vi "openMotor.vi"(3 "S/N Motor":string(combo)) -> (0 "Device":refnum<k24>, 1 ".NET Refnum out":refnum<k24>)   [LabVIEW 2014]
doc: "André Romero\nandretec@ifsc.usp.br"
uses:
  C:/user-Lab/AndreTec/GITs/andretec/Thorlabs-Vector-Move/kinesisTec/Kinesis/Thorlabs.MotionControl.Controls.dll
  kinesisTec/Kinesis/Thorlabs.MotionControl.Controls.dll
  C:/user-Lab/AndreTec/GITs/andretec/Thorlabs-Vector-Move/kinesisTec/Kinesis/Thorlabs.MotionControl.TCube.DCServoCLI.dll
  kinesisTec/Kinesis/Thorlabs.MotionControl.TCube.DCServoCLI.dll
panel:
  out "error out":errorcluster
  in  ".NET Refnum in":refnum<k24>(container)
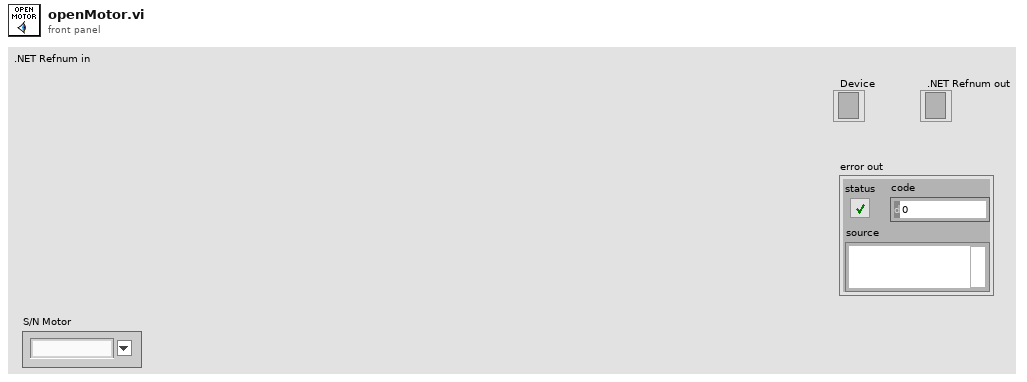
[diagram p1: front panel]
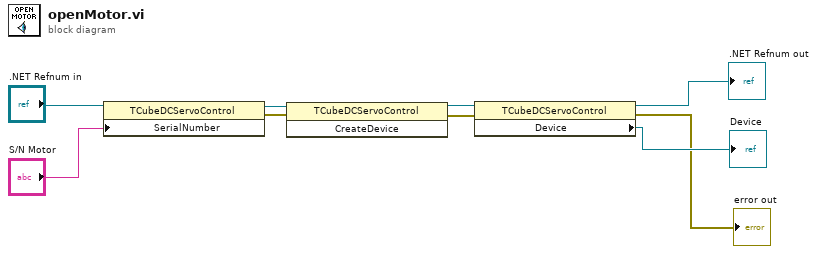
[diagram p0: block diagram]
diagram:
  n1 = property class="TCubeDCServoControl"(reference=".NET Refnum in", "SerialNumber"="S/N Motor") -> (reference out=w7:refnum<k24>, error out=w3:errorcluster)  [unwired: 1 in]
  n2 = invoke class="TCubeDCServoControl" method="CreateDevice"(reference=w7, error in=w3) -> (reference out=w8:refnum<k24>, error out=w2:errorcluster)  [unwired: 1 in, 1 out]
  n3 = property class="TCubeDCServoControl"(reference=w8, error in=w2) -> (reference out=→".NET Refnum out":refnum<k24>, error out=→"error out":errorcluster, "Device"=→"Device":refnum<k24>)
